vi "Parse GSV Sentence.vi"(8 "error in (no error)":errorcluster, 11 "GSV sentence":string) -> (0 "error out":errorcluster, 3 "GSV data":T1 {"satellite data"."data"."signal to noise ratio" min=0 max=99; "satellite data"."data"."azimuth (deg)" min=0 max=359; "satellite data"."data"."elevation (deg)" min=0 max=90; "number of satellites in view"."number of satellites" min=0; "sentence index"."index" min=0; "number of sentences for full data"."number of sentences" min=0})   [LabVIEW 2017, in "NMEA API.lvlib"]
doc: "Returns data contained in a particular type of NMEA sentence. The input sentence you specify must include valid NMEA formatting and end with a carriage return and line feed, or \\r\\n. You must manually select the polymorphic instance to use."
uses:
  <vilib>/robotics/Protocols/NMEA/NMEA API.lvlib
  <vilib>/robotics/Protocols/NMEA/typedefs/GSV Data.ctl
  <vilib>/robotics/Utilities/NI_Robotics Utilities.lvlib
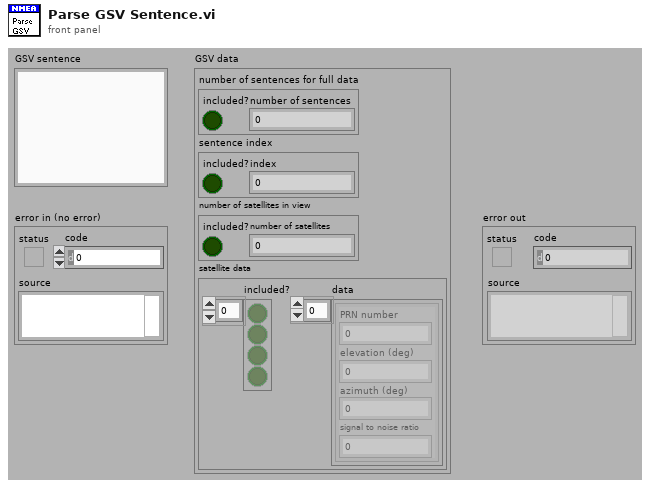
[diagram p1: front panel]
types:
  T1 = typedef "NMEA API.lvlib/GSV Data.ctl" = cluster{"number of sentences for full data":cluster{"included?":bool, "number of sentences":i8}, "sentence index":cluster{"included?":bool, "index":i8}, "number of satellites in view":cluster{"included?":bool, "number of satellites":i8}, "satellite data":cluster{"included?":bool[], "data":cluster{"PRN number":i32, "elevation (deg)":i32, "azimuth (deg)":i32, "signal to noise ratio":i32}[]}}
  T2 = cluster{"Included?":bool[], "Satellite Data":cluster{"PRN Number":i32, "Elevation (deg)":i32, "Azimuth (deg)":i32, "Signal to Noise Ratio":i32}[]}
  T3 = cluster{"PRN Number":i32, "Elevation (deg)":i32, "Azimuth (deg)":i32, "Signal to Noise Ratio":i32}
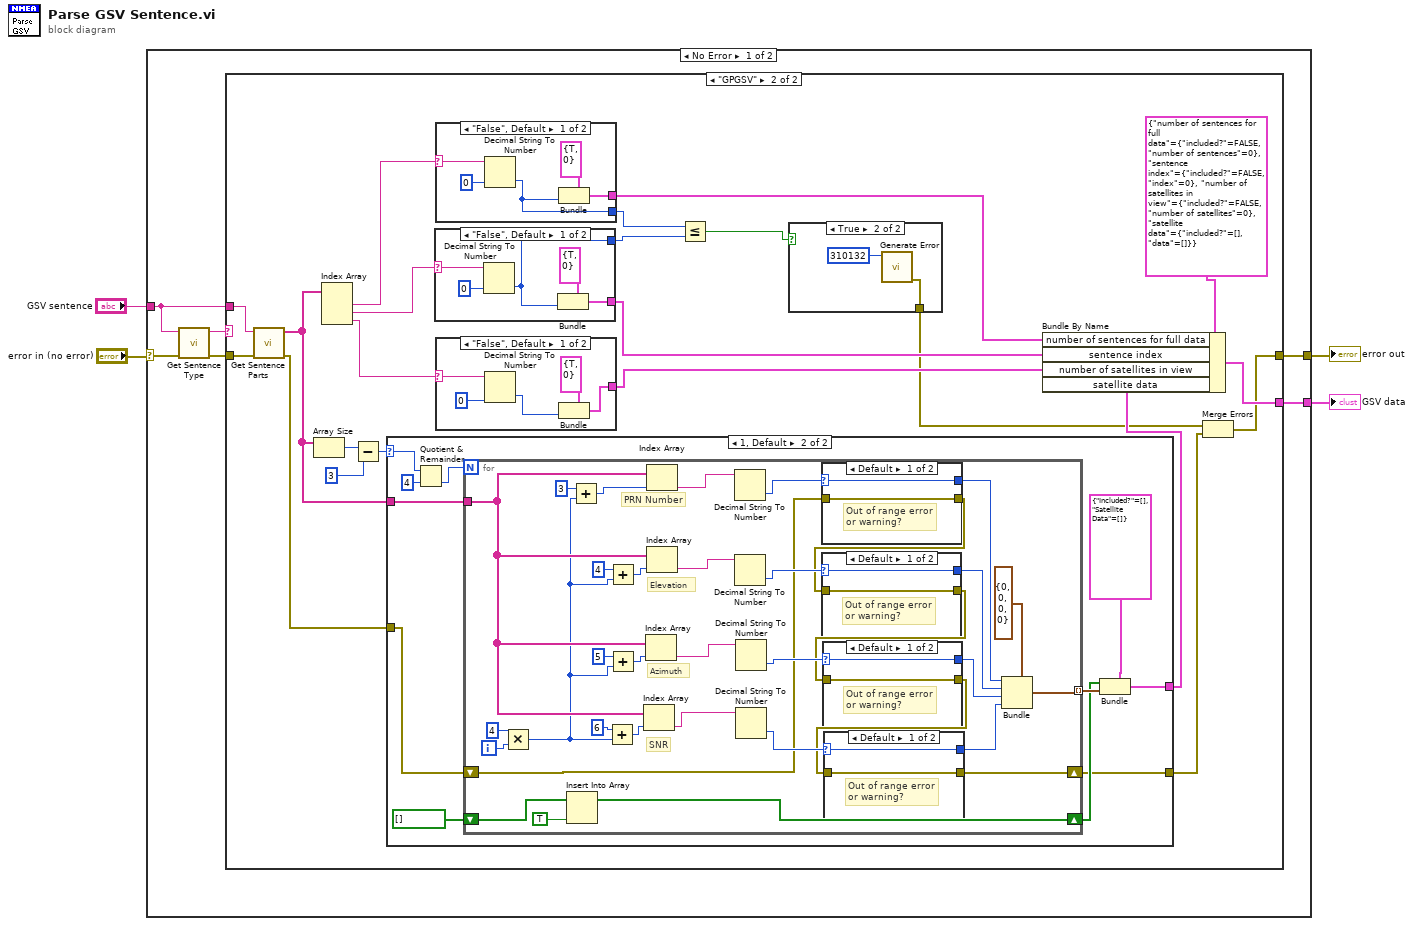
[diagram p0: block diagram]
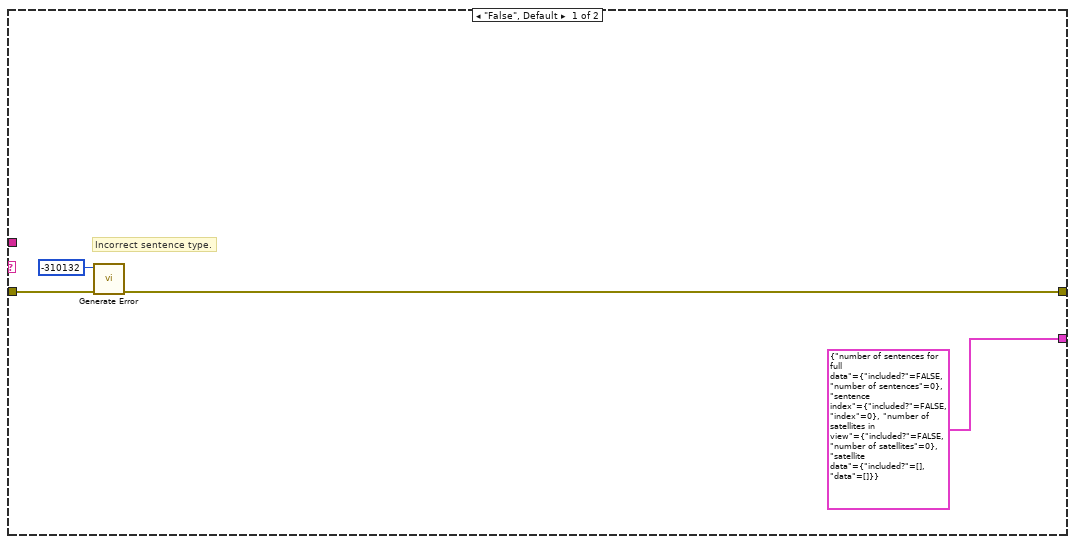
[diagram p2: hidden frame]
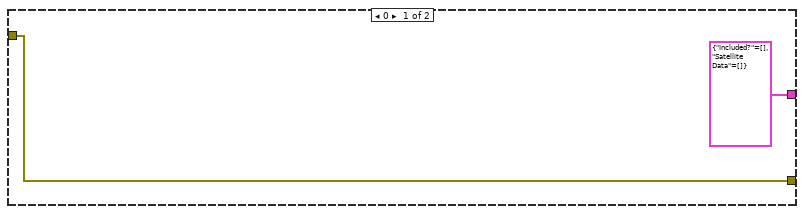
[diagram p4: hidden frame]
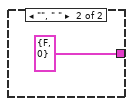
[diagram p9: hidden frame]
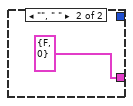
[diagram p10: hidden frame]
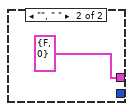
[diagram p11: hidden frame]
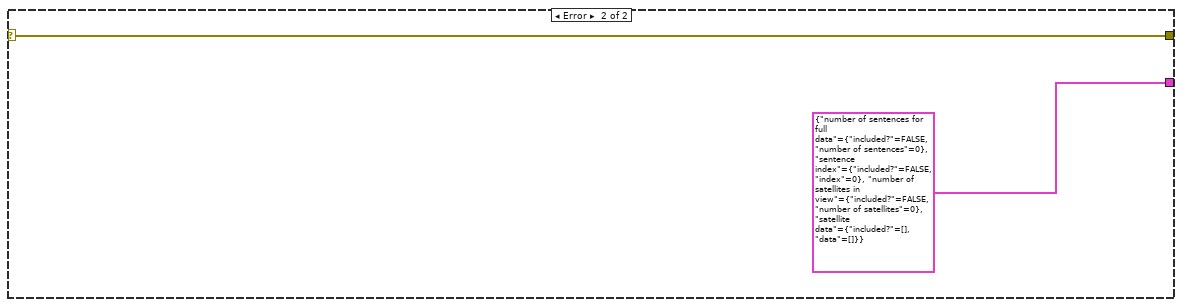
[diagram p12: hidden frame]
diagram:
  n1 = case shown="No Error" "error in (no error)" {
    selector: "error in (no error)" -> [w8 w121]
    tunnel: [w10 T1 {"number of sentences for full data"={"included?"=FALSE, "number of sentences"=0}, "sentence index"={"included?"=FALSE, "index"=0}, "number of satellites in view"={"included?"=FALSE, "number of satellites"=0}, "satellite data"={"included?"=[], "data"=[]}} ("GSV Data")] -> w4
    tunnel: [w9 w121] -> w3
    tunnel: "GSV sentence" -> [w6 _]
    frame No Error {
      n2 = call <vilib>:"Get Sentence Type.vi"("error in (no error)"=w8, "sentence"=w6) -> ("error out"=w7:errorcluster, "sentence type"=w5:string)  [unwired: 1 in, 7 out]
      n3 = case shown="\"GPGSV\"" w5 {
        tunnel: w7 -> [w12 w36]
        tunnel: w6 -> [_ w23]
        tunnel: [T1 {"number of sentences for full data"={"included?"=FALSE, "number of sentences"=0}, "sentence index"={"included?"=FALSE, "index"=0}, "number of satellites in view"={"included?"=FALSE, "number of satellites"=0}, "satellite data"={"included?"=[], "data"=[]}} ("GSV Data") w35] -> w10
        tunnel: [w11 w15] -> w9
        frame "False", Default {
          # "Incorrect sentence type."
          n4 = call <vilib>:"Generate Error.vi"("error in (no error)"=w12, "code"=-310132) -> ("error out"=w11:errorcluster)  [unwired: 9 in]
        }
        frame "GPGSV" {
          n5 = call <vilib>:"Get Sentence Parts.vi"("error in (no error)"=w36, "sentence"=w23) -> ("error out"=w21:errorcluster, "sentence data"=w22:string[])  [unwired: 1 in, 7 out]
          n6 = Array Size(array=w22) -> (size(s)=w27:i32)
          n7 = Index Array(array=w22) -> (element #1=w33:string, element #2=w31:string, element #3=w30:string)  [unwired: 3 in]
          n8 = Subtract(x=w27, y=3) -> (x-y=w25:i32)
          n9 = case shown="1, Default" w25 {
            selector: w25 -> [_ w48]
            tunnel: w22 -> [_ w49]
            tunnel: [T2 {"Included?"=[], "Satellite Data"=[]} ("Satellite Data") w45] -> w24
            tunnel: w21 -> [w39 w42]
            tunnel: [w39 w41] -> w17
            frame 0 {
            }
            frame 1, Default {
              n10 = Quotient & Remainder(x=w48, y=4) -> (floor(x/y)=w50:i32)  [unwired: 1 out]
              n11 = for {
                N: w50 -> [_]
                tunnel: [w81] -> w47 mode=indexing
                tunnel: w49 -> [w77]
                shift-right: [w66] -> w43
                shift-left: bool[] [] ("Included?") -> [w68]
                shift-right: [w56] -> w41
                shift-left: w42 -> [w60]
                i -> [w79]
                # "SNR"
                # "Azimuth"
                # "Elevation"
                # "PRN Number"
                n12 = Multiply(x=4, y=w79) -> (x*y=w69:i32)
                n13 = Insert Into Array(array=w68, new element=TRUE ("new element/subarray")) -> (w66:bool[])  [unwired: 1 in]
                n14 = Add(x=3, y=w69) -> (x+y=w76:i32)
                n15 = Add(x=6, y=w69) -> (x+y=w70:i32)
                n16 = Add(x=4, y=w69) -> (x+y=w74:i32)
                n17 = Add(x=5, y=w69) -> (x+y=w72:i32)
                n18 = Index Array(array=w77, index=w70) -> (element=w82:string)
                n19 = Index Array(array=w77, index=w72) -> (element=w83:string)
                n20 = Index Array(array=w77, index=w76) -> (element=w85:string)
                n21 = Index Array(array=w77, index=w74) -> (element=w84:string)
                n22 = Decimal String To Number(string=w85) -> (number=w64:i32)  [unwired: 2 in, 1 out]
                n23 = Decimal String To Number(string=w84) -> (number=w63:i32)  [unwired: 2 in, 1 out]
                n24 = Decimal String To Number(string=w83) -> (number=w62:i32)  [unwired: 3 out]
                n25 = Decimal String To Number(string=w82) -> (number=w61:i32)  [unwired: 2 in, 1 out]
                n26 = case shown="Default" w64 {
                  selector: w64 -> [w98 w100]
                  tunnel: w60 -> [w99 w101]
                  tunnel: [w99 w101] -> w59
                  tunnel: [w98 w100] -> w55
                  frame Default {
                    # "Out of range error\nor warning?"
                  }
                  frame 0..32 {
                    # "Valid range"
                  }
                }
                n27 = case shown="Default" w63 {
                  selector: w63 -> [w94 w96]
                  tunnel: w59 -> [w95 w97]
                  tunnel: [w95 w97] -> w58
                  tunnel: [w94 w96] -> w54
                  frame Default {
                    # "Out of range error\nor warning?"
                  }
                  frame 0..90 {
                    # "Valid range"
                  }
                }
                n28 = case shown="Default" w62 {
                  selector: w62 -> [w90 w92]
                  tunnel: w58 -> [w91 w93]
                  tunnel: [w91 w93] -> w57
                  tunnel: [w90 w92] -> w53
                  frame Default {
                    # "Out of range error\nor warning?"
                  }
                  frame 0..359 {
                    # "Valid range"
                  }
                }
                n29 = case shown="Default" w61 {
                  selector: w61 -> [w86 w88]
                  tunnel: w57 -> [w87 w89]
                  tunnel: [w87 w89] -> w56
                  tunnel: [w86 w88] -> w52
                  frame Default {
                    # "Out of range error\nor warning?"
                  }
                  frame 0..99 {
                    # "Valid range"
                  }
                }
                n30 = Bundle(cluster=T3 {"PRN Number"=0, "Elevation (deg)"=0, "Azimuth (deg)"=0, "Signal to Noise Ratio"=0} ("Satellite 1 Data"), "PRN Number"=w55, "Elevation (deg)"=w54, "Azimuth (deg)"=w53, "Signal to Noise Ratio"=w52) -> (w81:T3)
              }
              n31 = Bundle(cluster=T2 {"Included?"=[], "Satellite Data"=[]} ("Satellite Data"), "Included?"=w43, "Satellite Data"=w47) -> (w45:T2)
            }
          }
          n32 = case shown="\"False\", Default" w31 {
            selector: w31 -> [w112 _]
            tunnel: [w110 cluster{"Valid?":bool, "# of Sentences":i8} {"Valid?"=FALSE, "# of Sentences"=0} ("Number of Sentences for Full Data")] -> w29
            tunnel: [w108 _] -> w19
            frame "False", Default {
              n33 = Decimal String To Number(string=w112, default (0L)=i8 0) -> (number=w108:i8)  [unwired: 2 out]
              n34 = Bundle(cluster=cluster{"Valid?":bool, "# of Sentences":i8} {"Valid?"=TRUE, "# of Sentences"=0} ("Number of Sentences for Full Data"), "# of Sentences"=w108) -> (w110:cluster{"Valid?":bool, "# of Sentences":i8})  [unwired: 1 out]
            }
            frame "", " " {
            }
          }
          n35 = case shown="\"False\", Default" w33 {
            selector: w33 -> [w118 _]
            tunnel: [w116 cluster{"Valid?":bool, "# of Sentences":i8} {"Valid?"=FALSE, "# of Sentences"=0} ("Number of Sentences for Full Data")] -> w32
            tunnel: [w114 _] -> w20
            frame "False", Default {
              n36 = Decimal String To Number(string=w118, default (0L)=i8 0) -> (number=w114:i8)  [unwired: 2 out]
              n37 = Bundle(cluster=cluster{"Valid?":bool, "# of Sentences":i8} {"Valid?"=TRUE, "# of Sentences"=0} ("Number of Sentences for Full Data"), "# of Sentences"=w114) -> (w116:cluster{"Valid?":bool, "# of Sentences":i8})  [unwired: 1 out]
            }
            frame "", " " {
            }
          }
          n38 = case shown="\"False\", Default" w30 {
            selector: w30 -> [w106 _]
            tunnel: [w103 cluster{"Valid?":bool, "# of Sentences":i8} {"Valid?"=FALSE, "# of Sentences"=0} ("Number of Sentences for Full Data")] -> w28
            frame "False", Default {
              n39 = Decimal String To Number(string=w106, default (0L)=i8 0) -> (number=w104:i8)  [unwired: 2 out]
              n40 = Bundle(cluster=cluster{"Valid?":bool, "# of Sentences":i8} {"Valid?"=TRUE, "# of Sentences"=0} ("Number of Sentences for Full Data"), "# of Sentences"=w104) -> (w103:cluster{"Valid?":bool, "# of Sentences":i8})  [unwired: 1 out]
            }
            frame "", " " {
            }
          }
          n41 = Less Or Equal?(x=w20, y=w19) -> (x <= y?=w18:bool)
          n42 = case shown="True" w18 {
            tunnel: [_ w37] -> w16
            frame False {
            }
            frame True {
              n43 = call <vilib>:"Generate Error.vi"("code"=310132) -> ("error out"=w37:errorcluster)  [unwired: 10 in]
            }
          }
          n44 = Bundle By Name(cluster=T1 {"number of sentences for full data"={"included?"=FALSE, "number of sentences"=0}, "sentence index"={"included?"=FALSE, "index"=0}, "number of satellites in view"={"included?"=FALSE, "number of satellites"=0}, "satellite data"={"included?"=[], "data"=[]}} ("GSV Data"), "number of sentences for full data"=w32, "sentence index"=w29, "number of satellites in view"=w28, "satellite data"=w24) -> (w35:T1)
          n45 = Merge Errors(w16, w17) -> (w15:errorcluster)
        }
      }
    }
    frame Error {
    }
  }
  "error out" <- w3
  "GSV data" <- w4
